vi "Get Windows Process Memory Usage.vi"() -> (3 "Memory Used By This Process (KB)":dbl)   [LabVIEW 2016]
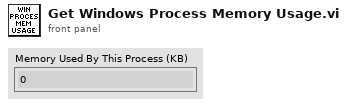
[diagram p1: front panel]
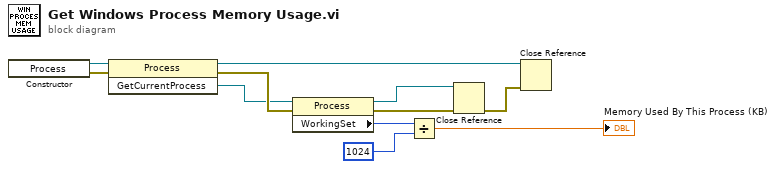
[diagram p0: block diagram]
diagram:
  n1 = constructor class="Process"() -> (reference out=w11:refnum<k24>, error out=w1:errorcluster)  [unwired: 3 in, 1 out]
  n2 = invoke class="Process" method="GetCurrentProcess"(reference=w11, error in=w1) -> (reference out=w8:refnum<k24>, error out=w10:errorcluster, "GetCurrentProcess"=w2:refnum<k24>)  [unwired: 1 in]
  n3 = property class="Process"(reference=w2, error in=w10) -> (reference out=w6:refnum<k24>, error out=w5:errorcluster, "WorkingSet"=w3:i32)
  n4 = Divide(x=w3, y=i64 1024) -> (x/y=→"Memory Used By This Process (KB)":dbl)
  n5 = Close Reference(reference=w6, error in (no error)=w5) -> (error out=w7:errorcluster)
  n6 = Close Reference(reference=w8, error in (no error)=w7) -> ()  [unwired: 1 out]
